vi "FPGAmain.vi"() -> ()   [LabVIEW 2019]
uses:
  <vilib>/rvi/eio/common/nirviEmuTemplateMethod_errors.vi
  <vilib>/rvi/Emulation/niFpgaGetClockAttributes.vi
  <vilib>/rvi/Emulation/niFpgaSctlEmulationGetInTimedLoop.vi
  <vilib>/rvi/Emulation/niFpgaEmulationReportErrorSimple.vi
  <vilib>/rvi/DataTransferAndStorage/Container/Common/niFpgaContainerExecOnDevCompGetState.vi
  <vilib>/rvi/Emulation/niFpgaEmulationIsFPGAContextNoSignature.vi
  <vilib>/rvi/errors/niFpgaSetErrorForExecOnDevCompSimple.vi
  <vilib>/rvi/eio/common/nirviEmuReportErrorAndStop.vi
  <vilib>/rvi/DataTransferAndStorage/Container/Common/niFpgaContainerGetUniqueNameForEmu.vi
  <vilib>/rvi/FIFO/Fifo_Resource/nirvififoEmulationSetSize.vi
  <vilib>/rvi/FIFO/Fifo_Resource/nirviFifoEmulationQueueMgr.vi
  <instcachedir>/0/nirviFifoEmulationQueueMgr_E5CAEC123FF24DC58D834DCA3CDAA9B5.lvgen/nirviFifoEmulationQueueMgr_E5CAEC123FF24DC58D834DCA3CDAA9B5_001.vi
  <vilib>/rvi/FIFO/Fifo_Resource/nirvififoEmulationDetermineInputValidOut.vi
  <vilib>/rvi/FIFO/Fifo_Resource/nirvififoEmulationCreateLock.vi
  <vilib>/rvi/Emulation/niFpgaProcessEmulError.vi
  <vilib>/rvi/FIFO/Fifo_Resource/nirvififoEmulationObtainLock.vi
  <vilib>/rvi/FIFO/Fifo_Resource/nirvififoEmulationReleaseLock.vi
  <vilib>/rvi/occurrence/nirviWaitOnOccurrenceBase.vi
  <vilib>/rvi/errors/nirviReportUnexpectedCaseInternalError.vi
  <vilib>/rvi/errors/nirviReportUnexpectedCaseInternalError (U32).vi
  <vilib>/Utility/error.llb/Clear Errors.vi
  <vilib>/rvi/interface/RandomDataEmulation/niFpgaRandomDataHandleErrors.vi
  <vilib>/rvi/Emulation/niFpgaCriticalErrorInLSC.vi
  <vilib>/eio/EIONode/EIONode.xnode
  <vilib>/rvi/DataTransferAndStorage/Container/XNode/niFpgaContainer.xnode
  <vilib>/rvi/FIFO/Fifo_Resource/niFpgaFifoEmulationRefIn.vi
  <vilib>/rvi/interface/RandomDataEmulation/nirviRandomDataFpgaReadWriteTemplate.vi
panel:
  out "Number of Elements to Read":u32
  out "FIFO from RT Overflow":bool
  out "Trq Calib Pt 1 (Amp)":sgl
  out "Trq Calib Pt 1 (ft-lbf)":sgl
  out "Trq Calib Pt 0 (Amp)":sgl
  out "Trq Calib Pt 0 (ft-lbf)":sgl
  out "Load 1 Zero":sgl
  out "Load 2 Zero":sgl
  out "Blk Calib Pt 1 (in)":sgl
  out "Blk Calib Pt 1 (Amp)":sgl
  out "Blk Calib Pt 0 (in)":sgl
  out "Blk Calib Pt 0 (Amp)":sgl
  out "Tach 1 Period (100 us)":u32
  out "Tach 2 Period (100 us)":u32
  out "Top Drive Torque":sgl
  out "Mod3-9203/AI0":sgl
  out "Total Thrust Force (lbf)":sgl
  out "Load 2: Force (lbf)":sgl
  out "Load 1: Force (lbf)":sgl
  out "Mod1-9237/AI1":sgl
  out "Mod1-9237/AI0":sgl
  out "Block Position (in)":sgl
  out "Mod3-9203/AI1":sgl
  out "FIFO to RT Overflow":bool
  # "FPGA Main"
  # "I/O and Data Processing"
  # "Thrust Force"
  # "Block Position"
  # "Top Drive Torque"
  # "Top Drive Tachometer"
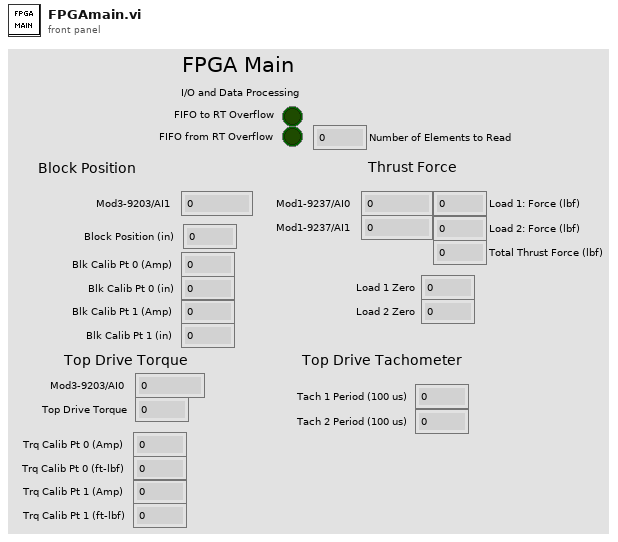
[diagram p1: front panel]
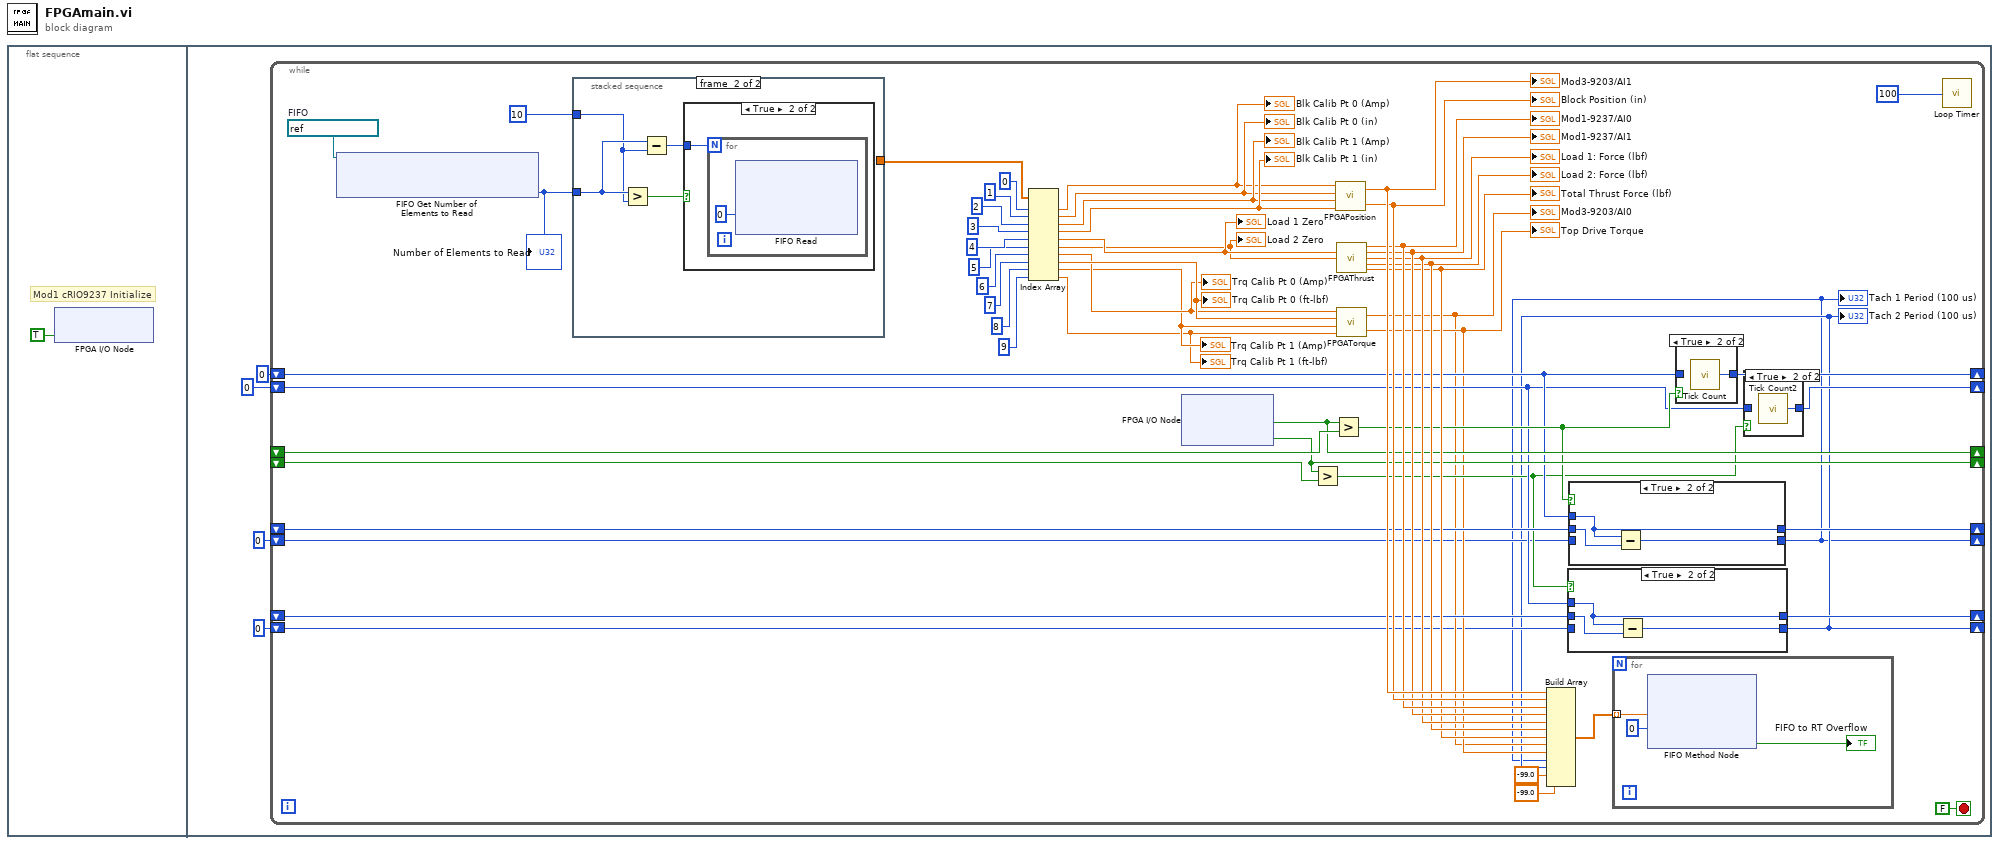
[diagram p0: block diagram]
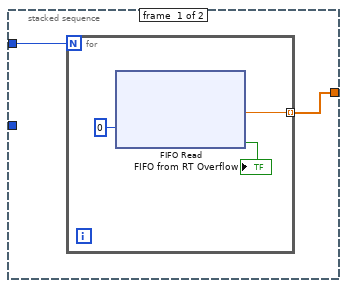
[diagram p2: hidden frame]
diagram:
  n1 = flat-sequence {
    frame #0 {
      # "Mod1 cRIO9237 Initialize"
      n2 = xnode "FPGA I/O Node"("Mod1/Start"=TRUE) -> ()  [unwired: 1 in, 1 out]
    }
    frame #1 {
      n3 = while {
        shift-right: [w51] -> _
        shift-left: u32 0 ("Tick Count(Ticks)") -> [w44]
        shift-right: [w49] -> _
        shift-left: _ -> [w50]
        shift-right: [w48] -> _
        shift-left: _ -> [w47]
        shift-right: [w46] -> _
        shift-left: u32 0 ("Tick Count(Ticks)") -> [w39]
        shift-right: [w43] -> _
        shift-left: _ -> [w42]
        shift-right: [w41] -> _
        shift-left: _ -> [w40]
        shift-right: [w33] -> _
        shift-left: u32 0 -> [w34]
        shift-right: [w32] -> _
        shift-left: u32 0 -> [w35]
        stop <- FALSE stop-if-true
        w9 = refnum<k21> "FIFO from RT"  # FIFO
        n4 = xnode ("FIFO Get Number of Elements to Read")("FIFO In"=w9) -> ("Number of Elements to Read"=w7:u32)  [unwired: 1 out]
        "Number of Elements to Read" <- w7
        n5 = stacked-sequence {
          tunnel: [w63 _] -> w8
          tunnel: w7 -> [_ w69]
          tunnel: i16 10 -> [w62 w68]
          frame #0 {
            n6 = for {
              N: w62 -> [_]
              tunnel: [w64] -> w63 mode=indexing
              n7 = xnode ("FIFO Read")("Timeout"=0) -> ("Element"=w64:sgl, "Timed Out?"=→"FIFO from RT Overflow":bool)  [unwired: 1 in, 1 out]
            }
          }
          frame #1 {
            n8 = Greater?(x=w69, y=w68) -> (0:w70:bool)
            n9 = Subtract(x=w69, y=w68) -> (x-y=w67:u32)
            n10 = case shown="True" w70 {
              tunnel: w67 -> [_ w71]
              frame False {
              }
              frame True {
                n11 = for {
                  N: w71 -> [_]
                  n12 = xnode ("FIFO Read")("Timeout"=0) -> ()  [unwired: 1 in, 3 out]
                }
              }
            }
          }
        }
        n13 = Index Array(array=w8, index #1=0 ("index"), index #2=1 ("index"), index #3=2 ("index"), index #4=3 ("index"), index #5=4 ("index"), index #6=5 ("index"), index #7=6 ("index"), index #8=7 ("index"), index #9=8 ("index"), index #10=9 ("index")) -> (element #1=w18:sgl, element #2=w19:sgl, element #3=w20:sgl, element #4=w21:sgl, element #5=w17:sgl, element #6=w12:sgl, element #7=w15:sgl, element #8=w16:sgl, element #9=w14:sgl, element #10=w13:sgl)
        "Blk Calib Pt 0 (in)" <- w19
        "Blk Calib Pt 0 (Amp)" <- w18
        "Blk Calib Pt 1 (in)" <- w21
        "Blk Calib Pt 1 (Amp)" <- w20
        "Load 2 Zero" <- w12
        "Load 1 Zero" <- w17
        "Trq Calib Pt 0 (ft-lbf)" <- w16
        "Trq Calib Pt 0 (Amp)" <- w15
        "Trq Calib Pt 1 (ft-lbf)" <- w13
        "Trq Calib Pt 1 (Amp)" <- w14
        n14 = xnode "FPGA I/O Node"() -> ("Mod2/DI0"=w49:bool, "Mod2/DI1"=w48:bool)  [unwired: 2 in, 2 out]
        n15 = Greater?(x=w48, y=w47) -> (0:w38:bool)
        n16 = Greater?(x=w49, y=w50) -> (0:w45:bool)
        n17 = call "FPGAPosition.vi"("Calib Pt 1 (in)"=w21, "Calib Pt 1 (amps)"=w20, "Calib Pt 0 (in)"=w19, "Calib Pt 0 (amps)"=w18) -> ("Block Position (in)"=w58:sgl, "Mod3-9203/AI1"=w59:sgl)
        "Mod3-9203/AI1" <- w59
        "Block Position (in)" <- w58
        n18 = call "FPGAThrust.vi"("Load 1: Zero"=w17, "Load 2: Zero"=w12) -> ("Mod1-9237/AI0"=w56:sgl, "Mod1-9237/AI1"=w55:sgl, "Load 1: Force (lbf)"=w54:sgl, "Load 2: Force (lbf)"=w53:sgl, "Total Thrust Force (lbf)"=w52:sgl)  [unwired: 9 in]
        "Mod1-9237/AI0" <- w56
        "Mod1-9237/AI1" <- w55
        "Load 1: Force (lbf)" <- w54
        "Load 2: Force (lbf)" <- w53
        "Total Thrust Force (lbf)" <- w52
        n19 = call "FPGATorque.vi"("Calib Pt 1 (ft-lbf)"=w13, "Calib Pt 1 (amps)"=w14, "Calib Pt 0 (ft-lbf)"=w16, "Calib Pt 0 (amps)"=w15) -> ("Top Drive Torque"=w37:sgl, "Mod3-9203/AI0"=w36:sgl)
        "Mod3-9203/AI0" <- w36
        "Top Drive Torque" <- w37
        n20 = case shown="True" w38 {
          tunnel: w39 -> [_ w76]
          tunnel: [w74 w76] -> w41
          tunnel: w40 -> [w74 w77]
          tunnel: [w73 w75] -> w33
          tunnel: w34 -> [w73 _]
          frame False {
          }
          frame True {
            n21 = Subtract(x=w76, y=w77) -> (x-y=w75:u32)
          }
        }
        "Tach 2 Period (100 us)" <- w33
        n22 = case shown="True" w45 {
          tunnel: w44 -> [_ w81]
          tunnel: [w79 w81] -> w43
          tunnel: w42 -> [w79 w82]
          tunnel: [w78 w80] -> w32
          tunnel: w35 -> [w78 _]
          frame False {
          }
          frame True {
            n23 = Subtract(x=w81, y=w82) -> (x-y=w80:u32)
          }
        }
        "Tach 1 Period (100 us)" <- w32
        n24 = Build Array(w59, w58, w56, w55, w54, w53, w52, w36, w37, w32, w33, sgl -99.0 ("element"), sgl -99.0 ("element")) -> (w57:sgl[])
        n25 = for {
          tunnel: w57 -> [w88] mode=indexing
          n26 = xnode ("FIFO Method Node")("Element"=w88, "Timeout"=0) -> ("Timed Out?"=→"FIFO to RT Overflow":bool)  [unwired: 1 in, 1 out]
        }
        n27 = case shown="True" w45 {
          tunnel: [w85 w86] -> w51
          tunnel: w44 -> [w85 _]
          frame False {
          }
          frame True {
            n28 = call "Tick Count"() -> ("Tick Count(mSec)"=w86:u32)
          }
        }
        n29 = case shown="True" w38 {
          tunnel: [w83 w84] -> w46
          tunnel: w39 -> [w83 _]
          frame False {
          }
          frame True {
            n30 = call "Tick Count2"() -> ("Tick Count(mSec)"=w84:u32)
          }
        }
        n31 = call "Loop Timer"("Count(uSec)"=u32 100 ("Count(mSec)")) -> ()  [unwired: 1 out]
      }
    }
  }
